vi "Write Conversion 2s Complement.vi"(11 "Set Data Input":i16) -> (3 "Coversion Data Output":i16)   [LabVIEW 2023, in "HardwareAbstractionLayer_LVOOP.lvlib" / "Modbus.lvclass"]
uses:
  Modbus.lvclass
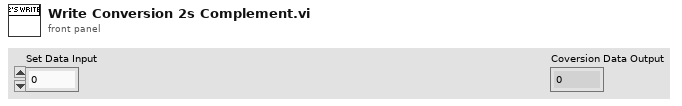
[diagram p1: front panel]
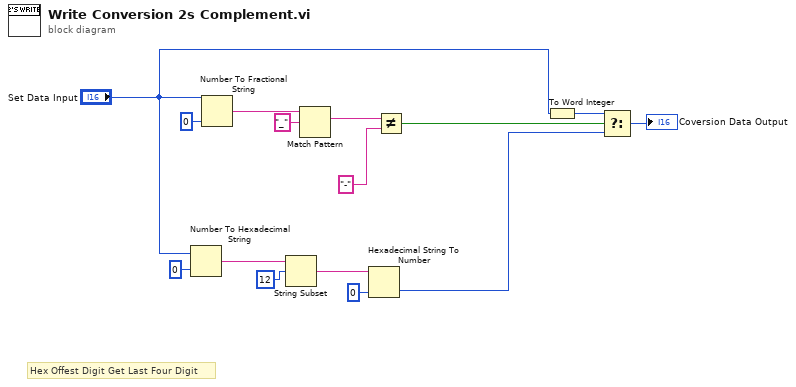
[diagram p0: block diagram]
diagram:
  # "Hex Offest Digit Get Last Four Digit"
  n1 = Number To Hexadecimal String(1:i16 0 ("width (-)"), 2:"Set Data Input") -> (0:w7:string)
  n2 = Number To Fractional String(number="Set Data Input", precision (6)=i16 0) -> (F-format string=w14:string)  [unwired: 2 in]
  n3 = String Subset(string=w7, offset (0)=12) -> (substring=w5:string)  [unwired: 1 in]
  n4 = Match Pattern(string=w14, regular expression="_") -> (match substring=w12:string)  [unwired: 1 in, 3 out]
  n5 = Hexadecimal String To Number(string=w5, default (0uL)=i16 0 ("default (0 U32)")) -> (number=w4:i16)  [unwired: 1 in, 1 out]
  n6 = Not Equal?(x=w12, y="-") -> (x != y?=w10:bool)
  n7 = To Word Integer(number="Set Data Input") -> (16bit integer=w3:i16)
  n8 = Select(t=w3, s=w10, f=w4) -> (s? t:f=→"Coversion Data Output":i16)
